vi "Rec Create - Command.vi"(5 "cache size (1)":i32=1 min=1, 6 "error in (no error)":errorcluster, 7 "cursor type":T1, 9 "command reference":T2) -> (0 "error out":errorcluster, 3 "recordset reference":T3)   [LabVIEW 2012, in "NI_Database_API_64.lvlib"]
doc: "Creates and initializes a new <B>Recordset</B> object which should be destroyed using the <B>Rec Destroy - Command</B> VI later."
uses:
  NI_Database_API_64.lvlib
  Rec DataMembers.ctl
  Connection.llb/Conn ObjectReference.ctl
  Rec ObjectReference.ctl
  Command.llb/Cmd ObjectReference.ctl
  Auxilliary.llb/DB Tools Cursor Type.ctl
panel:
  in  "ADODB._Recordset":refnum<k7>
  in  "default data":T4
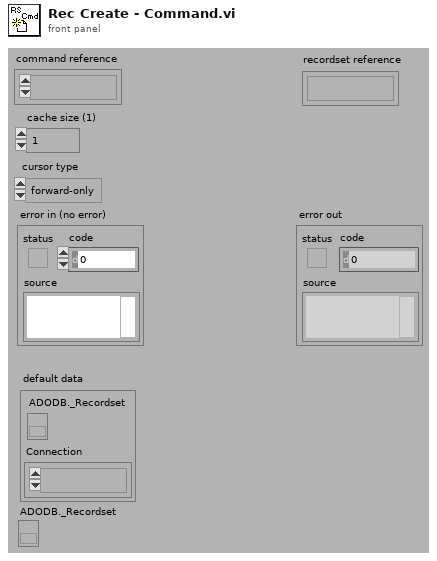
[diagram p1: front panel]
types:
  T1 = typedef "NI_Database_API_64.lvlib/DB Tools Cursor Type.ctl" = enum16{"forward-only", "keyset", "dynamic", "static"}
  T2 = typedef "NI_Database_API_64.lvlib/Cmd ObjectReference.ctl" = refnum<k1>
  T3 = typedef "NI_Database_API_64.lvlib/Rec ObjectReference.ctl" = refnum<k1>
  T4 = typedef "NI_Database_API_64.lvlib/Rec DataMembers.ctl" = cluster{"ADODB._Recordset":refnum<k7>, "Connection":T5}
  T5 = typedef "NI_Database_API_64.lvlib/Conn ObjectReference.ctl" = refnum<k1>
  T6 = typedef "NI_Database_API_64.lvlib/Cmd DataMembers.ctl" = cluster{"ADODB._Command":refnum<k7>, "Connection":T5}
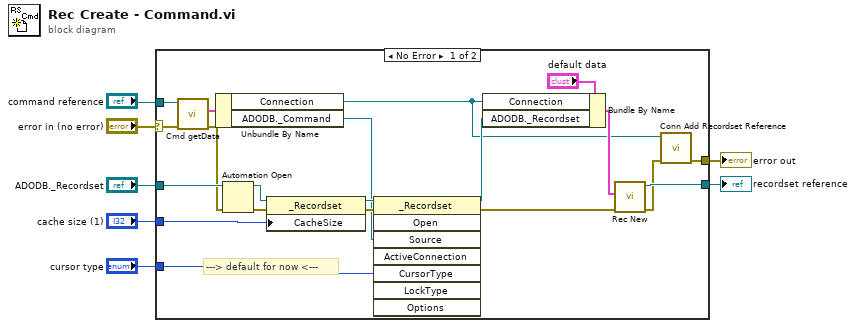
[diagram p0: block diagram]
diagram:
  n1 = case shown="No Error" "error in (no error)" {
    selector: "error in (no error)" -> [w12 w28]
    tunnel: [w27 _] -> w7
    tunnel: "command reference" -> [w22 _]
    tunnel: "ADODB._Recordset" -> [w11 _]
    tunnel: [w18 w28] -> w4
    tunnel: "cache size (1)" -> [w16 _]
    tunnel: "cursor type" -> [w15 _]
    frame No Error {
      # "---> default for now <---"
      n2 = call "Cmd getData.vi"("error in (no error)"=w12, "command reference"=w22) -> ("error out"=w8:errorcluster, "data"=w21:T6)  [unwired: 2 in, 2 out]
      n3 = Unbundle By Name(w21) -> ("Connection"=w19:T5, "ADODB._Command"=w13:refnum<k7>)
      n4 = Automation Open(error in (no error)=w8, Automation Refnum=w11) -> (Automation Refnum=w10:refnum<k7>, error out=w9:errorcluster)  [unwired: 2 in]
      n5 = property class="_Recordset"(reference=w10, error in=w9, "CacheSize"=w16) -> (reference out=w14:refnum<k7>, error out=w17:errorcluster)
      n6 = invoke class="_Recordset" method="Open"(reference=w14, error in=w17, "Source"=w13, "CursorType"=w15) -> (reference out=w25:refnum<k7>, error out=w23:errorcluster)  [unwired: 4 in, 6 out]
      n7 = Bundle By Name(cluster="default data", "Connection"=w19, "ADODB._Recordset"=w25) -> (w24:T4)
      n8 = call "Rec New.vi"("error in (no error)"=w23, "initial data"=w24) -> ("error out"=w20:errorcluster, "recordset reference"=w27:T3)  [unwired: 3 in, 1 out]
      n9 = call "Conn Add Recordset Reference.vi"("error in (no error)"=w20, "connection reference"=w19) -> ("error out"=w18:errorcluster)  [unwired: 9 in]
    }
    frame Error {
    }
  }
  "recordset reference" <- w7
  "error out" <- w4
